vi "DisplayLCD.vi"() -> ()   [LabVIEW 2015]
uses:
  <vilib>/Rock Robotics/WPI/SerialPort/WPI_SerialPortRef.ctl
panel:
  out "error out":errorcluster
  in  "Display string":string
  out "SerialPortRef 2":T1
  in  "error in (no error)":errorcluster
  in  "SerialPortRef":T1
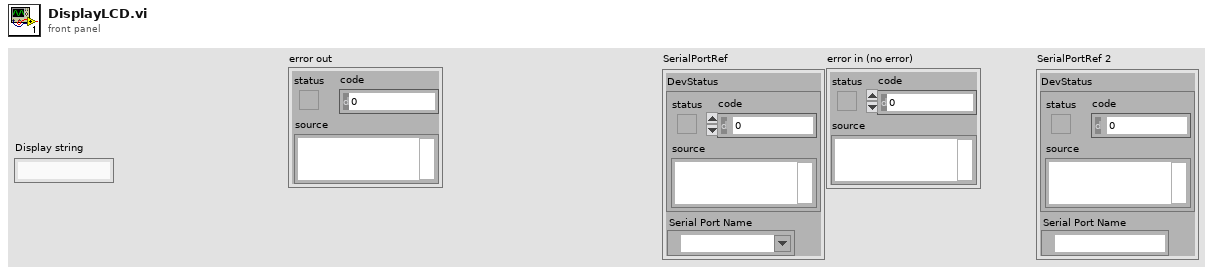
[diagram p1: front panel]
types:
  T1 = typedef "WPI_SerialPortRef.ctl" = cluster{"DevStatus":errorcluster, "Serial Port Name":refnum<visa-resource-name>}
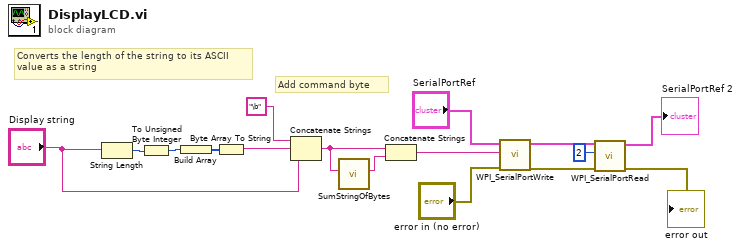
[diagram p0: block diagram]
diagram:
  # "Converts the length of the string to its ASCII \nvalue as a string"
  # "Add command byte"
  n1 = String Length(string="Display string") -> (length=w4:i32)
  n2 = To Unsigned Byte Integer(number=w4) -> (unsigned 8bit integer=w3:u8)
  n3 = Build Array(w3) -> (w2:u8[])
  n4 = Byte Array To String(unsigned byte array=w2) -> (string=w1:string)
  n5 = Concatenate Strings("\b" ("Buffer"), w1, "Display string") -> (w6:string)
  n6 = call "SumStringOfBytes.vi"("String Of Bytes"=w6) -> ("SumAsString"=w10:string)  [unwired: 10 in]
  n7 = Concatenate Strings(w6, w10) -> (w9:string)
  n8 = call <vilib>:"WPI_SerialPortWrite.vi"("error in (no error)"="error in (no error)", "Buffer"=w9, "SerialPortRef"="SerialPortRef") -> ("error out"=w13:errorcluster, "SerialPortRef"=w14:T1)  [unwired: 6 in, 1 out]
  n9 = call <vilib>:"WPI_SerialPortRead.vi"("error in (no error)"=w13, "Num Bytes to Read"=u32 2, "SerialPortRef"=w14) -> ("error out"=→"error out":errorcluster, "SerialPortRef"=→"SerialPortRef 2":T1)  [unwired: 6 in, 1 out]
